vi "generate random measurement value.vi"(8 "error in (no error)":errorcluster) -> (0 "error out":errorcluster, 2 "Random Measurement Value (5 - 10)":dbl)   [LabVIEW 2019]
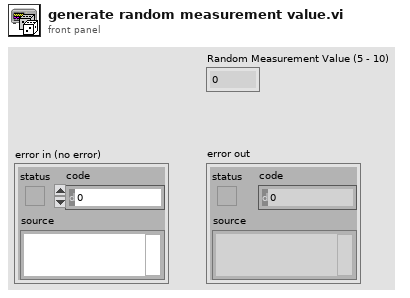
[diagram p1: front panel]
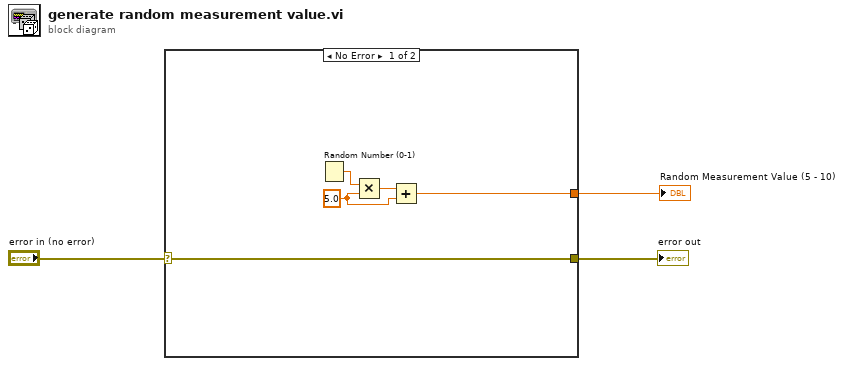
[diagram p0: block diagram]
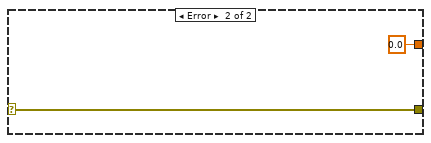
[diagram p2: hidden frame]
diagram:
  n1 = case shown="No Error" "error in (no error)" {
    selector: "error in (no error)" -> [w4 w10]
    tunnel: [w5 0.0] -> w3
    tunnel: [w4 w10] -> w1
    frame No Error {
      w8 = 5.0 ("number (0 to 1)")
      n2 = Random Number (0-1)() -> (number: 0 to 1=w6:dbl)
      n3 = Multiply(x=w6, y=w8) -> (x*y=w7:dbl)
      n4 = Add(x=w7, y=w8) -> (x+y=w5:dbl)
    }
    frame Error {
    }
  }
  "error out" <- w1
  "Random Measurement Value (5 - 10)" <- w3
